vi "SearchData.vi"(0 "ArrayIn":u8[](array[numeric]) format="0x%x") -> (1 "ArrayOut":u8[](array[numeric]) format="0x%x", 2 "Array1":u8[](array[numeric]) format="0x%x", 3 "Array2":u8[](array[numeric]) format="0x%x")   [LabVIEW 2011]
panel:
  # "从采集到的数据中获取自己需要的数据段"
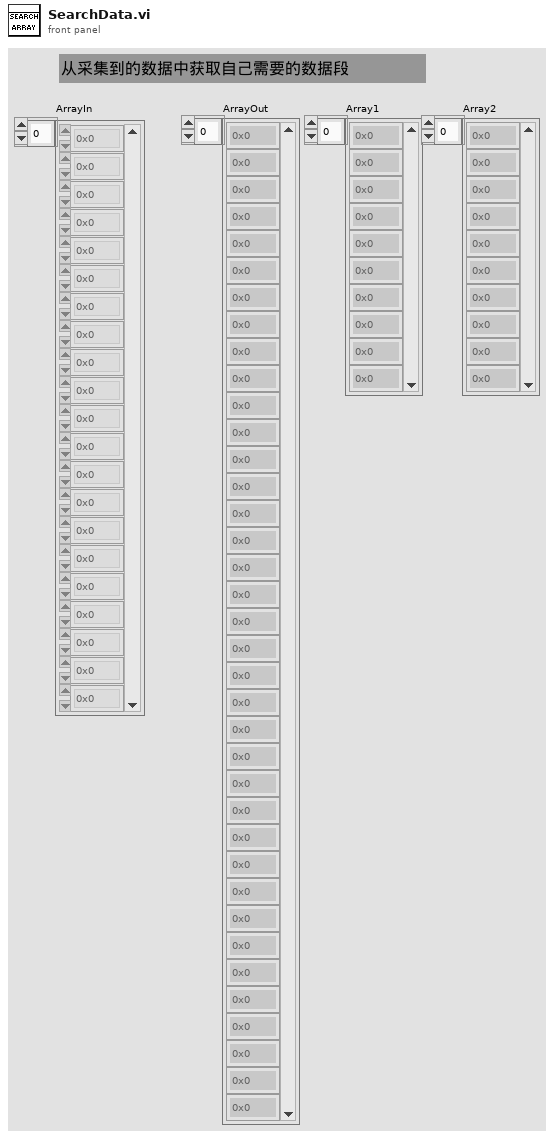
[diagram p1: front panel]
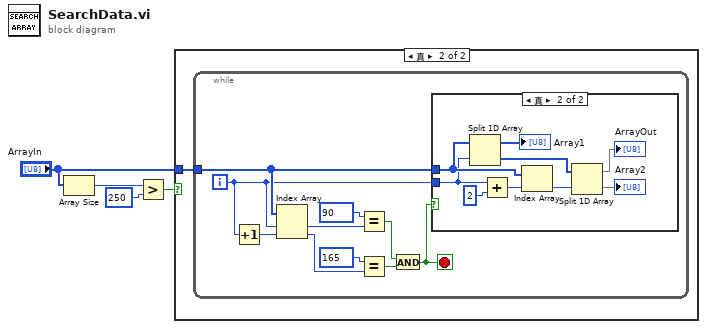
[diagram p0: block diagram]
diagram:
  n1 = Array Size(array="ArrayIn") -> (size(s)=w4:i32)
  n2 = Greater?(x=w4, y=250) -> (0:w2:bool)
  n3 = case shown="真" w2 {
    tunnel: "ArrayIn" -> [_ w5]
    frame False {
    }
    frame True {
      n4 = while {
        tunnel: w5 -> [w7]
        i -> [w6]
        stop <- w8 stop-if-true
        n5 = Increment(x=w6) -> (x+1=w15:i32)
        n6 = Index Array(array=w7, index #1=w6, index #2=w15) -> (element #1=w13:u8, element #2=w12:u8)
        n7 = Equal?(x=u8 90, y=w13) -> (x = y?=w10:bool)
        n8 = Equal?(x=u8 165, y=w12) -> (x = y?=w9:bool)
        n9 = And(x=w10, y=w9) -> (x .and. y?=w8:bool)
        n10 = case shown="真" w8 {
          tunnel: w7 -> [_ w23]
          tunnel: w6 -> [_ w22]
          frame False {
          }
          frame True {
            n11 = Split 1D Array(array=w23, index=w22) -> (first subarray=→"Array1":u8[], second subarray=w24:u8[])
            n12 = Add(x=w22, y=2) -> (x+y=w20:i32)
            n13 = Index Array(array=w23, index=w20) -> (element=w19:u8)
            n14 = Split 1D Array(array=w24, index=w19) -> (first subarray=→"ArrayOut":u8[], second subarray=→"Array2":u8[])
          }
        }
      }
    }
  }
